vi "VariableAnalogOutput.vi"() -> ()   [LabVIEW 2020]
uses:
  Control 1.ctl
  <vilib>/DAQmx/write.llb/DAQmx Write (Analog DBL 1Chan 1Samp).vi
  <vilib>/DAQmx/create/channels.llb/DAQmx Create Channel (AO-Voltage-Basic).vi
  <vilib>/DAQmx/miscellaneous.llb/DAQmx Fill In Error Info.vi
panel:
  in  "stop":bool
  in  "Min":dbl min=-10.0 max=9.0
  in  "Max":dbl min=-1.0 max=10.0
  in  "Slide":dbl(slide) min=0.0 max=0.0 scale=-2.0..10.0
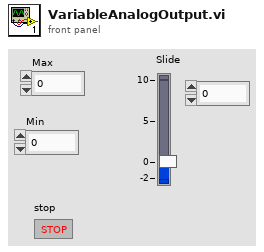
[diagram p1: front panel]
types:
  T1 = typedef "Control 1.ctl" = enum16{"Initialize", "Check UI", "Stop"}
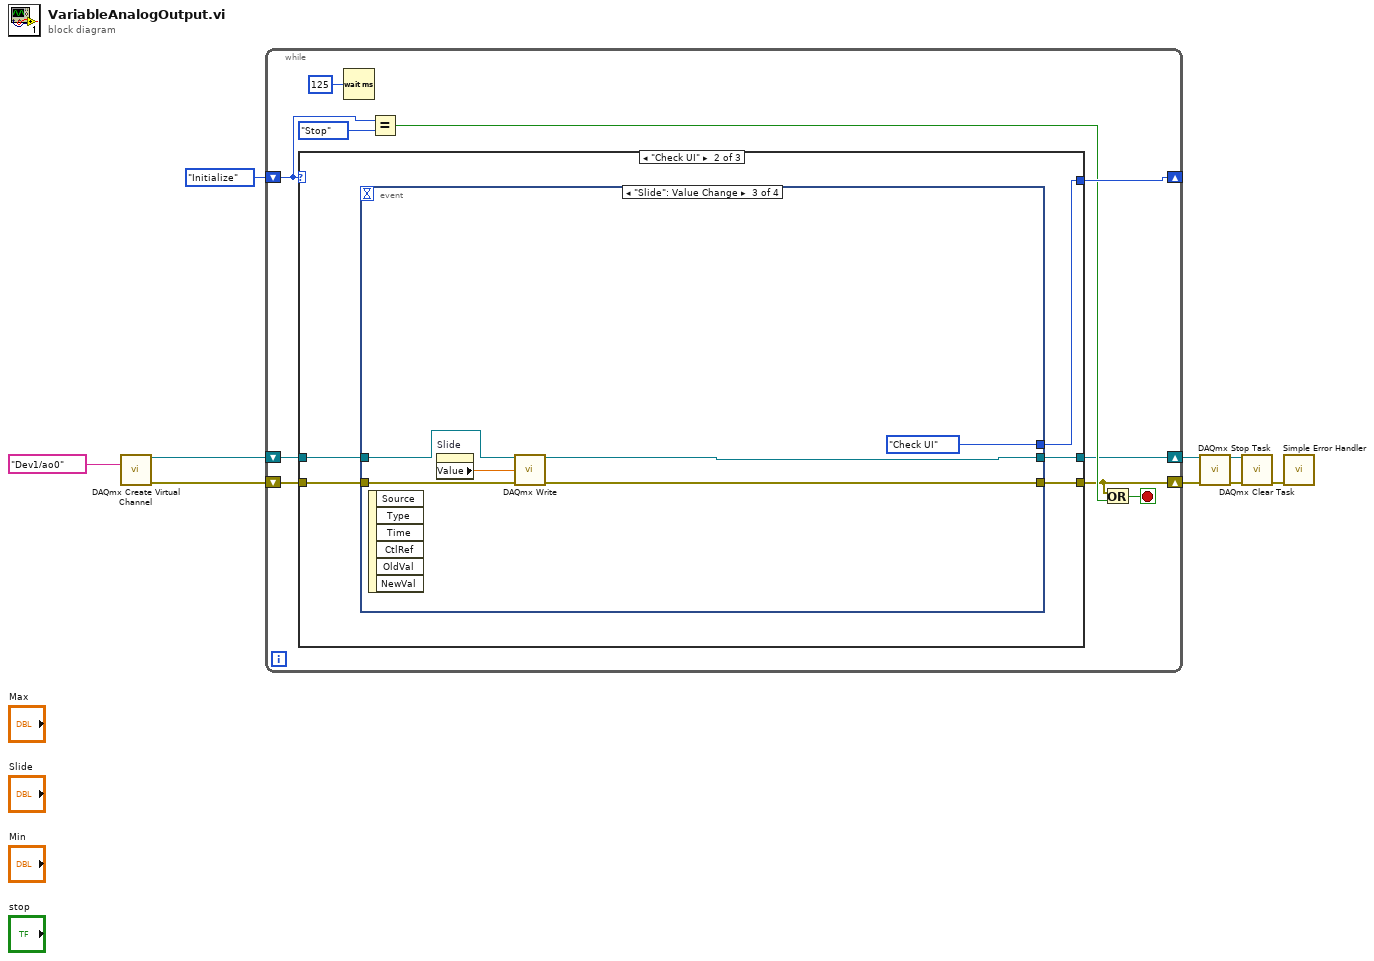
[diagram p0: block diagram]
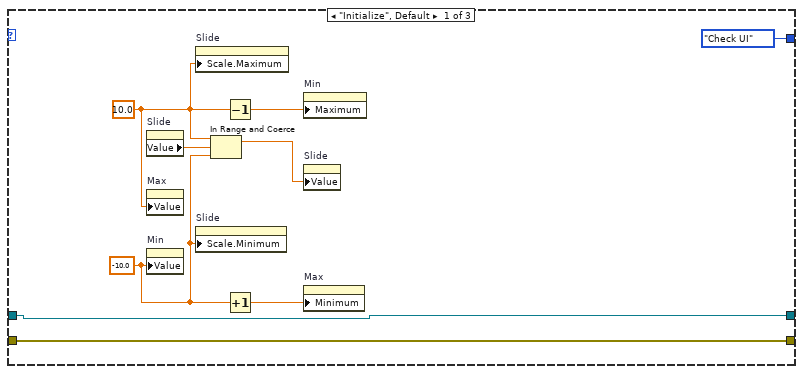
[diagram p2: hidden frame]
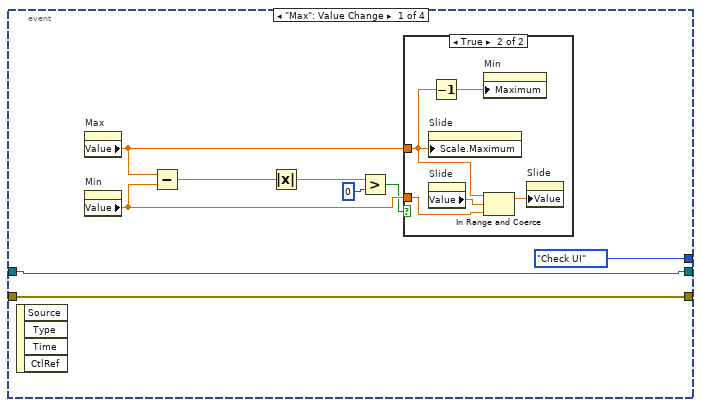
[diagram p3: hidden frame]
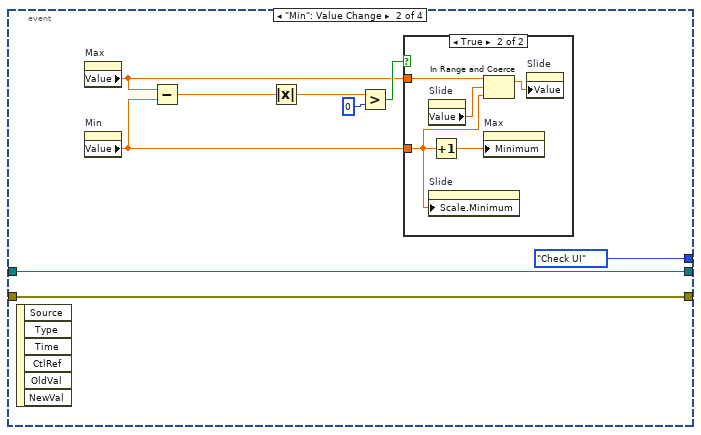
[diagram p5: hidden frame]
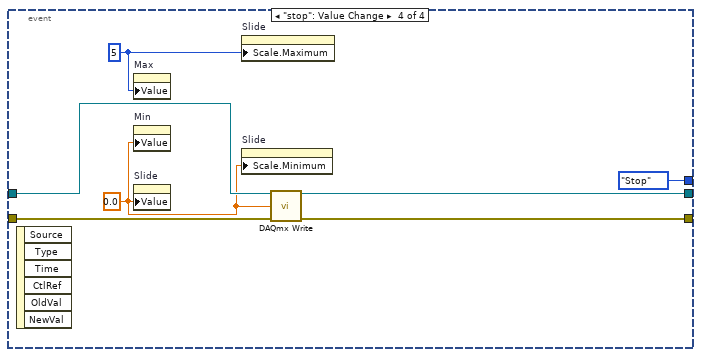
[diagram p7: hidden frame]
diagram:
  n1 = call-poly <vilib>:"DAQmx Create Virtual Channel.vi"("physical channels"=tag "Dev1/ao0") -> ("task out"=w8:refnum<k21>, "error out"=w6:errorcluster)  [unwired: 13 in]
  n2 = while {
    shift-right: [w19] -> _
    shift-left: Control_1."Initialize" -> [w17]
    shift-right: [w13] -> w3
    shift-left: w6 -> [w15]
    shift-right: [w11] -> w2
    shift-left: w8 -> [w16]
    stop <- w12 stop-if-true
    n3 = case shown="\"Check UI\"" w17 {
      tunnel: [Control_1."Check UI" w33 _] -> w19
      tunnel: w16 -> [w27 w32 w76]
      tunnel: [w26 w31 w75] -> w13
      tunnel: w15 -> [w26 w30 w75]
      tunnel: [w27 w29 w76] -> w11
      frame "Initialize", Default {
        w22 = -10.0 ("Min")
        w23 = 10.0 ("Max")
        n4 = property on="Slide" class="Slide (strict)"() -> ("Value"=w25:dbl)  [unwired: 2 in, 2 out]
        n5 = property on="Max" class="DigNum (strict)"("Value"=w23) -> ()  [unwired: 2 in, 2 out]
        n6 = property on="Min" class="DigNum (strict)"("Value"=w22) -> ()  [unwired: 2 in, 2 out]
        n7 = property on="Slide" class="Slide (strict)"("Scale.Maximum"=w23) -> ()  [unwired: 2 in, 2 out]
        n8 = property on="Slide" class="Slide (strict)"("Scale.Minimum"=w22) -> ()  [unwired: 2 in, 2 out]
        n9 = In Range and Coerce(upper limit=w23, x=w25, lower limit=w22) -> (coerced(x)=w24:dbl)  [unwired: 1 out]
        n10 = Decrement(x=w23) -> (x-1=w21:dbl)
        n11 = Increment(x=w22) -> (x+1=w20:dbl)
        n12 = property on="Min" class="DigNum (strict)"("Maximum"=w21) -> ()  [unwired: 2 in, 2 out]
        n13 = property on="Slide" class="Slide (strict)"("Value"=w24) -> ()  [unwired: 2 in, 2 out]
        n14 = property on="Max" class="DigNum (strict)"("Minimum"=w20) -> ()  [unwired: 2 in, 2 out]
      }
      frame "Check UI" {
        n15 = event shown="[2] \"Slide\": Value Change" {
          selector: _ -> [_ _ _ _]
          dyn-events: _ -> [_ _ _ _]
          timeout: _ -> [_ _ _ _]
          tunnel: [Control_1."Check UI" Control_1."Check UI" Control_1."Check UI" Control_1."Stop"] -> w33
          tunnel: w32 -> [w41 w55 w66 w73]
          tunnel: [w41 w55 w65 w70] -> w29
          tunnel: [w40 w54 w64 w71] -> w31
          tunnel: w30 -> [w40 w54 w63 w72]
          event "Max": Value Change {
            n16 = event-data() -> ()  [unwired: 1 in, 4 out]
            n17 = property on="Max" class="DigNum (strict)"() -> ("Value"=w38:dbl)  [unwired: 2 in, 2 out]
            n18 = property on="Min" class="DigNum (strict)"() -> ("Value"=w39:dbl)  [unwired: 2 in, 2 out]
            n19 = Subtract(x=w38, y=w39) -> (x-y=w37:dbl)
            n20 = Absolute Value(x=w37) -> (abs(x)=w34:dbl)
            n21 = Greater?(x=w34, y=0) -> (0:w35:bool)
            n22 = case shown="True" w35 {
              tunnel: w39 -> [_ w47]
              tunnel: w38 -> [_ w44]
              frame False {
              }
              frame True {
                n23 = property on="Slide" class="Slide (strict)"("Scale.Maximum"=w44) -> ()  [unwired: 2 in, 2 out]
                n24 = property on="Slide" class="Slide (strict)"() -> ("Value"=w46:dbl)  [unwired: 2 in, 2 out]
                n25 = Decrement(x=w44) -> (x-1=w43:dbl)
                n26 = property on="Min" class="DigNum (strict)"("Maximum"=w43) -> ()  [unwired: 2 in, 2 out]
                n27 = In Range and Coerce(upper limit=w44, x=w46, lower limit=w47) -> (coerced(x)=w45:dbl)  [unwired: 1 out]
                n28 = property on="Slide" class="Slide (strict)"("Value"=w45) -> ()  [unwired: 2 in, 2 out]
              }
            }
          }
          event "Min": Value Change {
            n29 = event-data() -> ()  [unwired: 1 in, 6 out]
            n30 = property on="Max" class="DigNum (strict)"() -> ("Value"=w50:dbl)  [unwired: 2 in, 2 out]
            n31 = property on="Min" class="DigNum (strict)"() -> ("Value"=w49:dbl)  [unwired: 2 in, 2 out]
            n32 = Subtract(x=w50, y=w49) -> (x-y=w53:dbl)
            n33 = Absolute Value(x=w53) -> (abs(x)=w48:dbl)
            n34 = Greater?(x=w48, y=0) -> (0:w52:bool)
            n35 = case shown="True" w52 {
              tunnel: w50 -> [_ w61]
              tunnel: w49 -> [_ w57]
              frame False {
              }
              frame True {
                n36 = property on="Slide" class="Slide (strict)"() -> ("Value"=w59:dbl)  [unwired: 2 in, 2 out]
                n37 = property on="Slide" class="Slide (strict)"("Scale.Minimum"=w57) -> ()  [unwired: 2 in, 2 out]
                n38 = Increment(x=w57) -> (x+1=w58:dbl)
                n39 = In Range and Coerce(upper limit=w61, x=w59, lower limit=w57) -> (coerced(x)=w60:dbl)  [unwired: 1 out]
                n40 = property on="Max" class="DigNum (strict)"("Minimum"=w58) -> ()  [unwired: 2 in, 2 out]
                n41 = property on="Slide" class="Slide (strict)"("Value"=w60) -> ()  [unwired: 2 in, 2 out]
              }
            }
          }
          event "Slide": Value Change {
            n42 = event-data() -> ()  [unwired: 1 in, 6 out]
            n43 = property on="Slide" class="Slide (strict)"() -> ("Value"=w67:dbl)  [unwired: 2 in, 2 out]
            n44 = call-poly <vilib>:"DAQmx Write.vi"("task/channels in"=w66, "data"=w67, "error in"=w63) -> ("task out"=w65:refnum<k21>, "error out"=w64:errorcluster)  [unwired: 10 in, 1 out]
          }
          event "stop": Value Change {
            w68 = 5
            w69 = 0.0 ("Slide")
            n45 = event-data() -> ()  [unwired: 1 in, 6 out]
            n46 = property on="Max" class="DigNum (strict)"("Value"=w68) -> ()  [unwired: 2 in, 2 out]
            n47 = property on="Min" class="DigNum (strict)"("Value"=w69) -> ()  [unwired: 2 in, 2 out]
            n48 = property on="Slide" class="Slide (strict)"("Value"=w69) -> ()  [unwired: 2 in, 2 out]
            n49 = property on="Slide" class="Slide (strict)"("Scale.Maximum"=w68) -> ()  [unwired: 2 in, 2 out]
            n50 = property on="Slide" class="Slide (strict)"("Scale.Minimum"=w69) -> ()  [unwired: 2 in, 2 out]
            n51 = call-poly <vilib>:"DAQmx Write.vi"("task/channels in"=w73, "data"=w69, "error in"=w72) -> ("task out"=w70:refnum<k21>, "error out"=w71:errorcluster)  [unwired: 10 in, 1 out]
          }
        }
      }
      frame "Stop" {
      }
    }
    n52 = Wait (ms)(milliseconds to wait=u32 125) -> ()  [unwired: 1 out]
    n53 = Equal?(x=w17, y=Control_1."Stop") -> (x = y?=w14:bool)
    n54 = Or(x=w13, y=w14) -> (x .or. y?=w12:bool)
  }
  n55 = call <vilib>:"DAQmx Stop Task.vi"("task/channels in"=w2, "error in"=w3) -> ("task out"=w5:refnum<k21>, "error out"=w4:errorcluster)  [unwired: 12 in]
  n56 = call <vilib>:"DAQmx Clear Task.vi"("task in"=w5, "error in"=w4) -> ("error out"=w1:errorcluster)  [unwired: 13 in]
  n57 = call <vilib>:"Simple Error Handler.vi"("error in (no error)"=w1) -> ()  [unwired: 4 in, 5 out]
